vi "CPP-Pitot.vi"(4 "Scan Period":dbl format="%.2f", 5 "Previous Scan Value":dbl format="%.2f", 6 "Present scan array":dbl[](array[numeric]) format="%.2f", 7 "Value to Output":dbl format="%.2f", 8 "Ch Description":T1={"Ch Name"="Tunnel3:Pressures:", "Type"="", "Function"=enum."Analogue Input", "Ch State"=enum."On", "Calibration type"=enum."Raw", "A"=30.0, "B"=10.0, "C"=0.0, "D"=0.0, "Comments"="", "Address"={"Main"=0, "Ch."=0, "Sub"=0, "Port Name"=""}, "String"="", "Duty"=65535} {"Duty" format="%.0b"; "D" format="%#_5g"; "C" format="%#_5g"; "B" format="%#_5g"; "A" format="%#_5g"}, 9 "Ch names":string[](array[string])) -> (0 "Scan comment":string, 1 "Output":dbl=0.0037402657506766107)   [LabVIEW 2015]
doc: "Wrapper for CPP-ZerosMaintenance.vi\nChannels Names should have the format \"Tunnel#:Pressures:\" (e.g. Tunnel1:Pressures: or Tunnel3:Pressures:). A = SecondsToMonitor (intervall to determine if tunnel has been off long enough and to inspect zero drift. B = SecondsToAverage (averaging interval for transducer zeros)."
uses:
  ADAM Client/Sub VIs/ADAM Controls/Ch_description_ADAM.ctl
  ADAM Client/Sub VIs/ADAM Controls/Module_type_ADAM.ctl
  ADAM Client/Sub VIs/ADAM Controls/Function_ADAM.ctl
  ADAM Client/Sub VIs/ADAM Controls/Channel_State.ctl
  ADAM Client/Sub VIs/ADAM Controls/Calib_type_ADAM.ctl
  ADAM Client/Sub VIs/ADAM Controls/Address.ctl
  Anemometry/Anemometry Sub Vis/Globals/Preference_global.vi
panel:
  in  "Ch names 3":string[](array[string])
  in  "Ch names 2":string[](array[string])
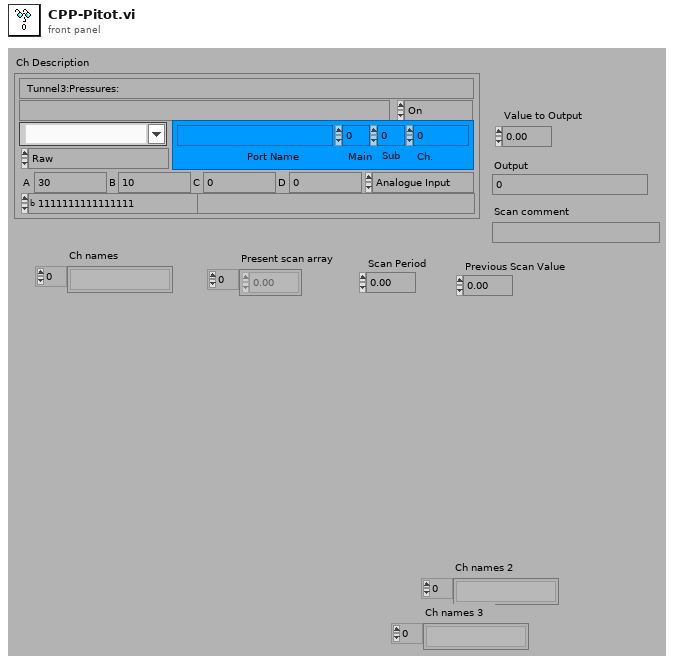
[diagram p1: front panel]
types:
  T1 = typedef "Ch_description_ADAM.ctl" = cluster{"Ch Name":string, "Type":T2, "Function":T3, "Ch State":T4, "Calibration type":T5, "A":dbl, "B":dbl, "C":dbl, "D":dbl, "Comments":string, "Address":T6, "String":string, "Duty":u16}
  T2 = typedef "Module_type_ADAM.ctl" = string
  T3 = typedef "Function_ADAM.ctl" = enum16{"Analogue Input", "Digital Input", "Event counter", "Event rate", "Analogue Output", "Digital Output", "Relay Output"}
  T4 = typedef "Channel_State.ctl" = enum16{"On", "Off", "Always On", "Always Off"}
  T5 = typedef "Calib_type_ADAM.ctl" = enum16{"Raw", "Bx + A", "Cx^2 + Bx + A", "Dx^3 + Cx^2 + Bx + A", "In Band", "Hi-Tec Q", "Hi-Tec M_dot", "Text"}
  T6 = typedef "Address.ctl" = cluster{"Main":i32, "Ch.":i32, "Sub":i32, "Port Name":string}
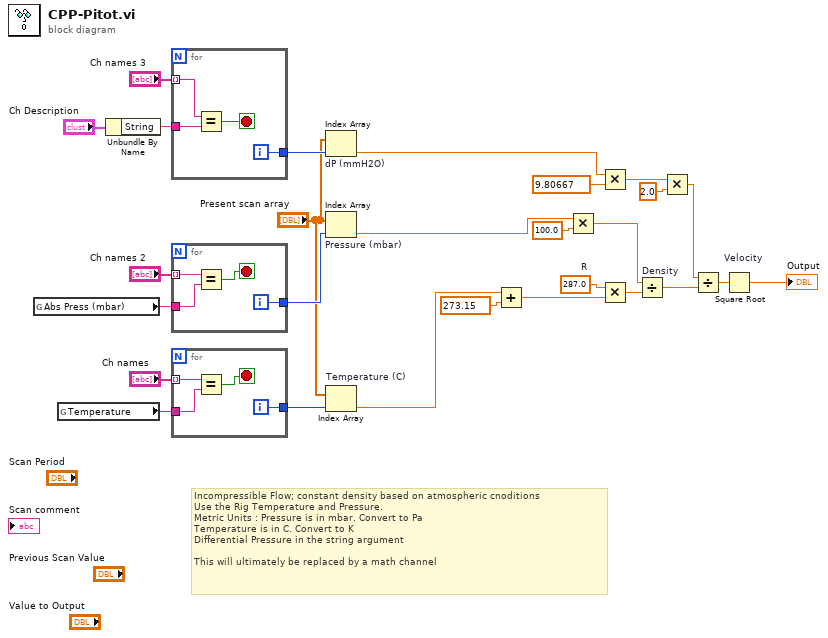
[diagram p0: block diagram]
diagram:
  w17 = 287.0  # R
  # "Incompressible Flow; constant density based on atmospheric cnoditions\nUse the Rig Temperature and Pressure. \nMetric Units : Pressure is in mbar. Convert to Pa\nTemperature is in C. Convert to K\nDifferential Pressure in the string argument\n\nThis will ultimately be replaced by a math channel"
  n1 = global read "Preference_global.vi" "Abs Press (mbar)"() -> (w22:string)
  n2 = global read "Preference_global.vi" "Temperature"() -> (w26:string)
  n3 = Unbundle By Name("Ch Description") -> ("String"=w10:string)
  n4 = for {
    tunnel: "Ch names 3" -> [w31] mode=indexing
    tunnel: w10 -> [w30]
    tunnel: [w28] -> w11
    i -> [w28]
    stop <- w29 stop-if-true
    n5 = Equal?(x=w31, y=w30) -> (x = y?=w29:bool)
  }
  n6 = for {
    tunnel: "Ch names 2" -> [w35] mode=indexing
    tunnel: w22 -> [w34]
    tunnel: [w32] -> w23
    i -> [w32]
    stop <- w33 stop-if-true
    n7 = Equal?(x=w35, y=w34) -> (x = y?=w33:bool)
  }
  n8 = for {
    tunnel: "Ch names" -> [w39] mode=indexing
    tunnel: w26 -> [w38]
    tunnel: [w36] -> w25
    i -> [w36]
    stop <- w37 stop-if-true
    n9 = Equal?(x=w39, y=w38) -> (x = y?=w37:bool)
  }
  n10 = Index Array "dP (mmH2O)"(array="Present scan array", index=w11) -> (element=w9:dbl)
  n11 = Index Array "Pressure (mbar)"(array="Present scan array", index=w23) -> (element=w21:dbl)
  n12 = Index Array "Temperature (C)"(array="Present scan array", index=w25) -> (element=w19:dbl)
  n13 = Add(x=w19, y=273.15) -> (x+y=w16:dbl)
  n14 = Multiply(x=w21, y=100.0) -> (x*y=w15:dbl)
  n15 = Multiply(x=w9, y=9.80667) -> (x*y=w6:dbl)
  n16 = Multiply(x=w17, y=w16) -> (x*y=w14:dbl)
  n17 = Divide "Density"(x=w15, y=w14) -> (x/y=w3:dbl)
  n18 = Multiply(x=w6, y=2.0) -> (x*y=w4:dbl)
  n19 = Divide(x=w4, y=w3) -> (x/y=w2:dbl)
  n20 = Square Root "Velocity"(x=w2) -> (sqrt(x)=→"Output":dbl)
